vi "CalcAngles.vi"(10 "Shoulder Y":u8, 11 "Elbow X":u8) -> (2 "Shoulder Degrees":dbl format="%.2f", 3 "Elbow Degrees":dbl format="%.2f")   [LabVIEW 2018]
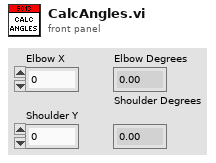
[diagram p1: front panel]
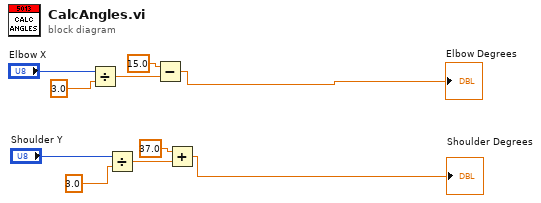
[diagram p0: block diagram]
diagram:
  n1 = Divide(x="Elbow X", y=3.0 ("Shoulder Y 3")) -> (x/y=w5:dbl)
  n2 = Divide(x="Shoulder Y", y=3.0 ("Shoulder Y 2")) -> (x/y=w9:dbl)
  n3 = Subtract(x=15.0 ("Shoulder Y 2"), y=w5) -> (x-y=→"Elbow Degrees":dbl)
  n4 = Add(x=37.0 ("Shoulder Y 2"), y=w9) -> (x+y=→"Shoulder Degrees":dbl)
